vi "(SubVI) Set Camera Image Format.vi"(4 "error in (no error)":errorcluster, 6 "Enum":enum16{"U8", "U16", "U12"}(ring), 7 "Refnum in":T1) -> (0 "error out":errorcluster, 3 "Refnum out":T1)   [LabVIEW 2014]
uses:
  <vilib>/userdefined/High Color/IMAQdx.ctl
  <resource>/objmgr/imaqdx.rc
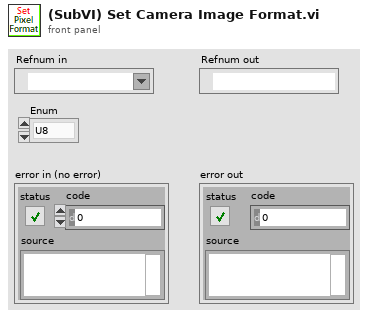
[diagram p1: front panel]
types:
  T1 = typedef "IMAQdx.ctl" = refnum<k21>
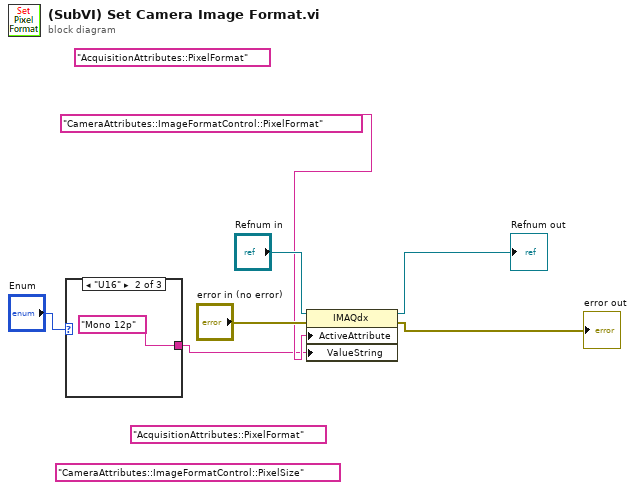
[diagram p0: block diagram]
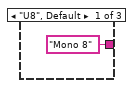
[diagram p2: hidden frame]
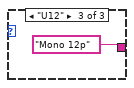
[diagram p3: hidden frame]
diagram:
  (unwired) "AcquisitionAttributes::PixelFormat"
  (unwired) "CameraAttributes::ImageFormatControl::PixelSize"
  (unwired) "AcquisitionAttributes::PixelFormat"
  n1 = case shown="\"U16\"" "Enum" {
    tunnel: ["Mono 8" "Mono 12p" "Mono 12p"] -> w1
    frame "U8", Default {
    }
    frame "U16" {
    }
    frame "U12" {
    }
  }
  n2 = property class="IMAQdx"(reference="Refnum in", error in="error in (no error)", "ActiveAttribute"="CameraAttributes::ImageFormatControl::PixelFormat", "ValueString"=w1) -> (reference out=→"Refnum out":T1, error out=→"error out":errorcluster)
